vi "Get Temperature.vi"(8 "error in (no error)":errorcluster, 11 "VIS-IR in":refnum<class "VIS-NIR.lvclass">) -> (0 "error out":errorcluster, 2 "Temperature":i32, 3 "VIS-IR out":refnum<class "VIS-NIR.lvclass">)   [LabVIEW 2015, in "VIS-NIR.lvclass"]
uses:
  VIS-NIR.lvclass
  Detector.lvclass
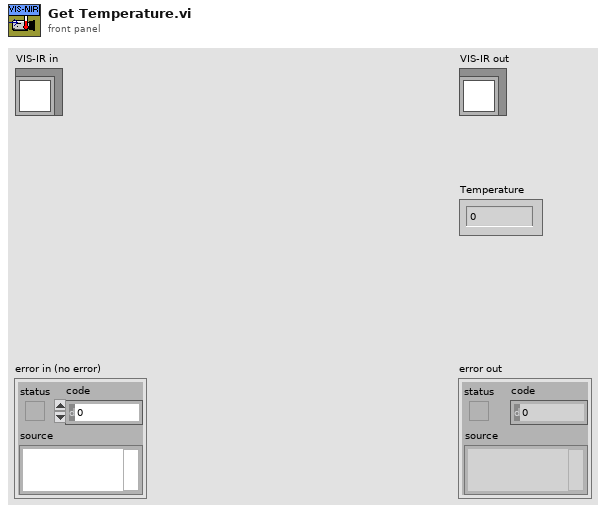
[diagram p1: front panel]
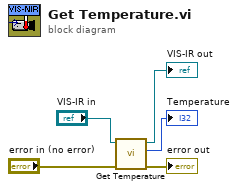
[diagram p0: block diagram]
diagram:
  n1 = call-parent "Get Temperature.vi"("error in (no error)"="error in (no error)", "Detector in"="VIS-IR in") -> ("error out"=→"error out":errorcluster, "Temperature"=→"Temperature":i32, "Detector out"=→"VIS-IR out":refnum<class "VIS-NIR.lvclass">)  [unwired: 7 in]
